vi "XIPIN_Video_Deinterlacer_3_00_a.vi"   [LabVIEW 2017]
doc: "Video Deinterlacer\n------------------------------------\n<b>Need License</b> : Yes\n<b>Interface</b> : AXI4 AXI4-Stream AXI4-Lite"
uses:
  <vilib>/rvi/XilinxIP/XIPIN_XNode/niFpgaXIPIN.xnode
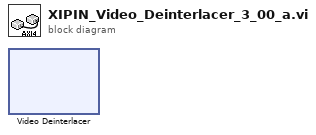
[diagram p0: block diagram]
diagram:
  n1 = xnode ("Video Deinterlacer")() -> ()
